vi "Operate.vi"(8 "error in (no error)":errorcluster, 11 "Add in":refnum<class "Add.lvclass">) -> (0 "error out":errorcluster, 2 "C":dbl, 3 "Add out":refnum<class "Add.lvclass">)   [LabVIEW 2021, in "Calculator.lvlib" / "Add.lvclass"]
doc: "This VI is a method for add class."
uses:
  Add.lvclass
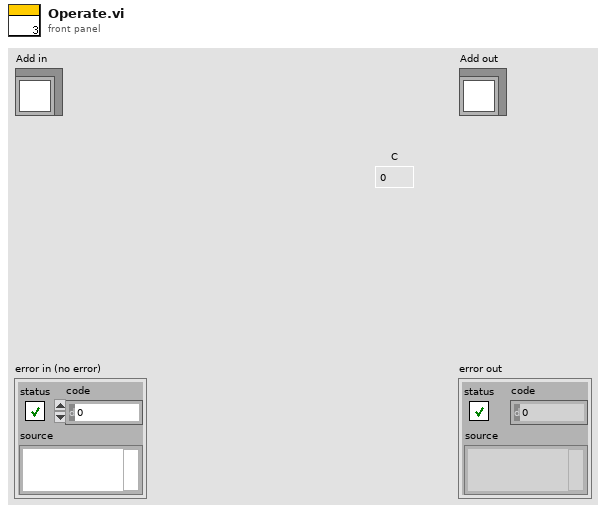
[diagram p1: front panel]
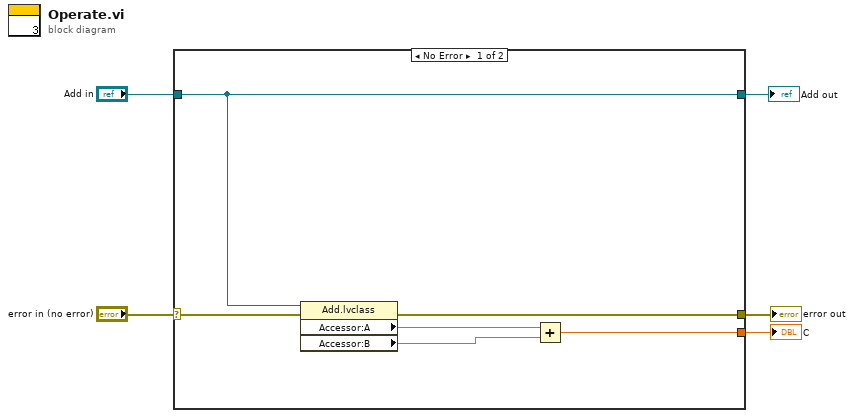
[diagram p0: block diagram]
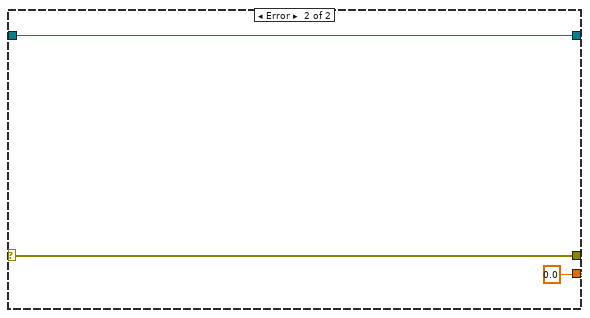
[diagram p2: hidden frame]
diagram:
  n1 = case shown="No Error" "error in (no error)" {
    selector: "error in (no error)" -> [w11 w14]
    tunnel: [w9 w14] -> w4
    tunnel: [w8 w13] -> w2
    tunnel: "Add in" -> [w8 w13]
    tunnel: [w10 0.0] -> w1
    frame No Error {
      n2 = property class="Add.lvclass"(reference=w8, error in=w11) -> (error out=w9:errorcluster, "Accessor:A"=w7:dbl, "Accessor:B"=w6:dbl)  [unwired: 1 out]
      n3 = Add(x=w7, y=w6) -> (x+y=w10:dbl)
    }
    frame Error {
    }
  }
  "error out" <- w4
  "Add out" <- w2
  "C" <- w1
